vi "Thorlabs_CCS_Test_Panel.vi"() -> ()   [LabVIEW 2021]
doc: "Instrument test panel"
uses:
  _Controls/Thorlabs_CCS_Detector_Info.ctl
  _Controls/Thorlabs_CCS_Configuration.ctl
panel:
  out "XY Graph":T1(graph)
  in  "Tab Control":enum32{"Detector", "Configuration", "Capture"}(tab)
  out "Detector":T2
  in  "Connect":bool
  in  "USB VISA Resource Name":string="USB0::0x1313::0x8089::M00463105::RAW"
  in  "Auto detect USB devices":bool
  in  "Configuration":T3={"Acquisition_Mode"=enum."Continuos", "Trigger_Source"=enum."Auto/Internal", "Integration_Time_[s]"=0.5}
  out "Period [s]":dbl
  out "Counter":i32
  in  "NbrLines":i32=-1 caption="NbrLines\n(-1=endless)" min=-2 max=1000000
  in  "Capture":bool
  out "# elements in queue":i32
  out "Error Message":string caption="Error Description"
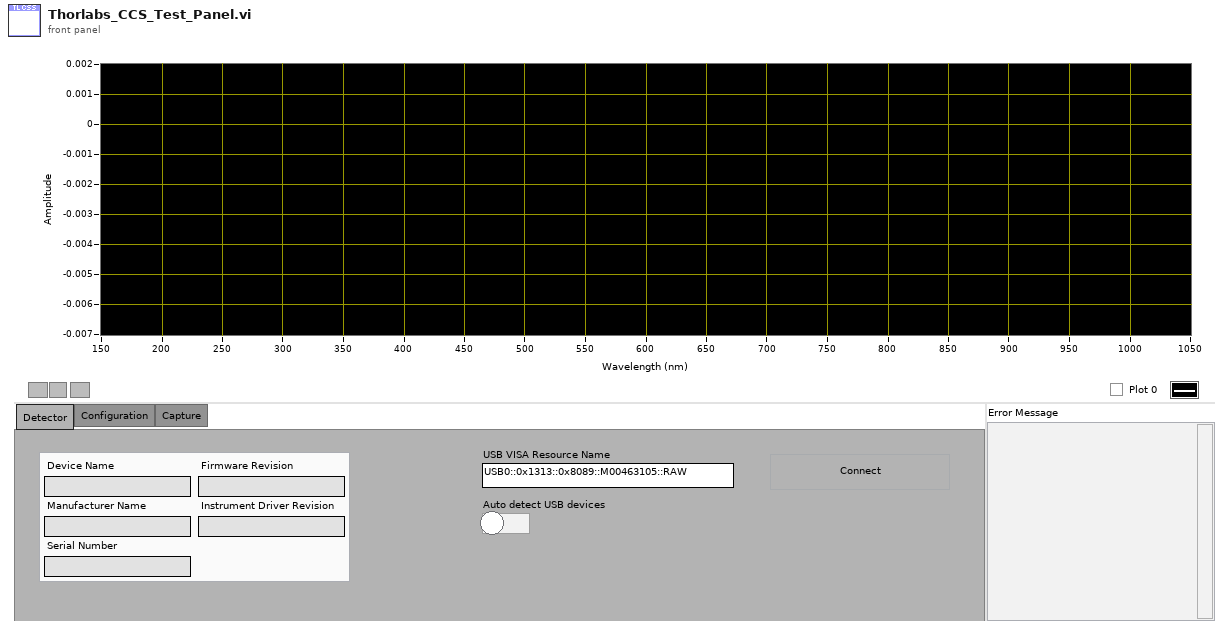
[diagram p1: front panel]
types:
  T1 = cluster{"Wavelength Data Array":dbl[], "Data":dbl[]}
  T2 = typedef "Thorlabs_CCS_Detector_Info.ctl" = cluster{"Device Name":string, "Manufacturer Name":string, "Serial Number":string, "Firmware Revision":string, "Instrument Driver Revision":string}
  T3 = typedef "Thorlabs_CCS_Configuration.ctl" = cluster{"Acquisition_Mode":enum16{"Single Scan", "Continuos"}, "Trigger_Source":enum16{"Auto/Internal", "External"}, "Integration_Time_[s]":dbl}
  T4 = cluster{"This VI":refnum<vi>, "Control":cluster{"Capture":refnum<vi>, "Tab Control":refnum<vi>, "NbrLines":refnum<vi>}, "Indicator":cluster{"Detector":refnum<vi>, "XY Graph":refnum<vi>}}
  T5 = enum32{"invalid app kind", "Development System", "Run Time System", "Student Edition", "Embedded LabVIEW", "Evaluation", "Custom"}
  T6 = enum8{"Enabled", "Disabled", "Disabled and Grayed Out"}
  T7 = enum32{"Page Enabled", "Page Disabled", "Page Disabled & Grayed"}
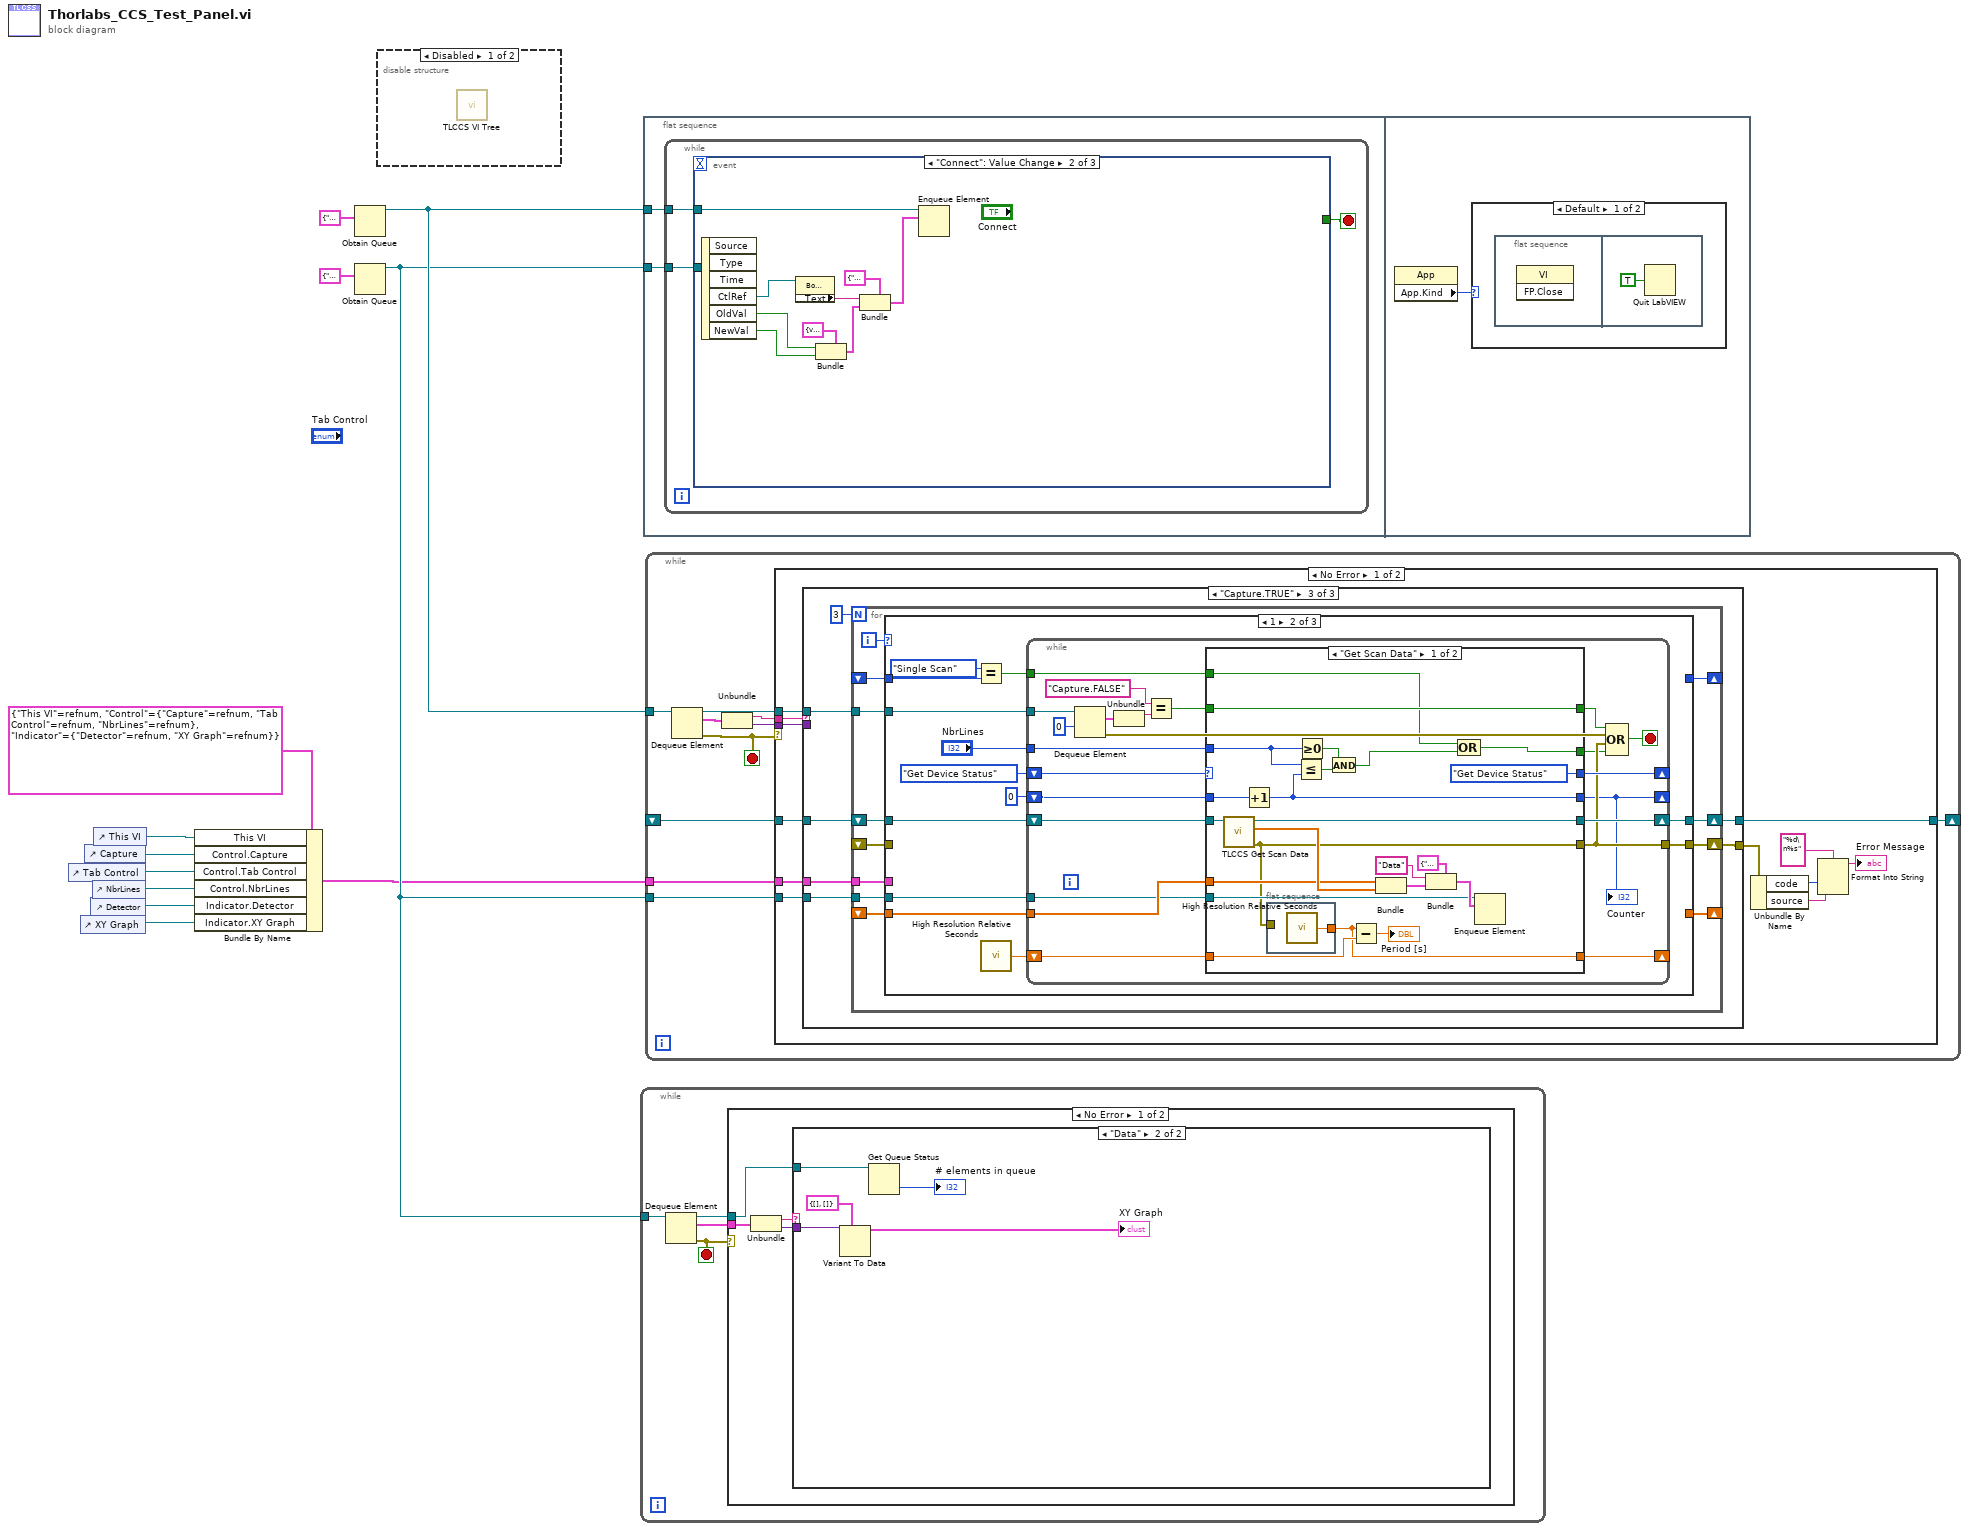
[diagram p0: block diagram]
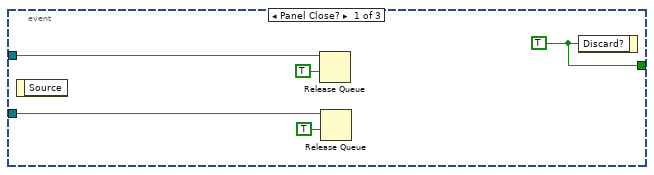
[diagram p5: hidden frame]
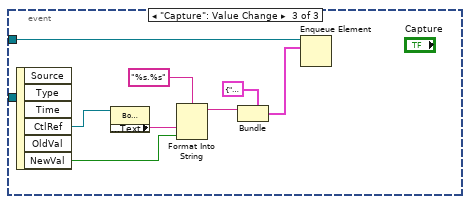
[diagram p6: hidden frame]
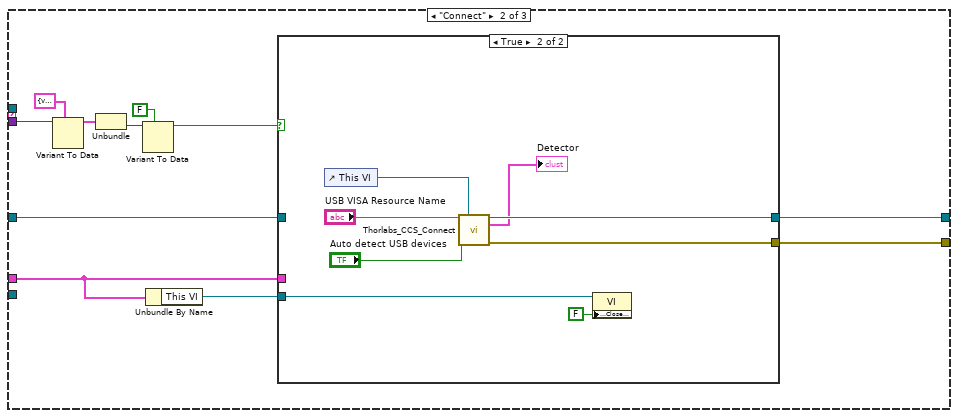
[diagram p9: hidden frame]
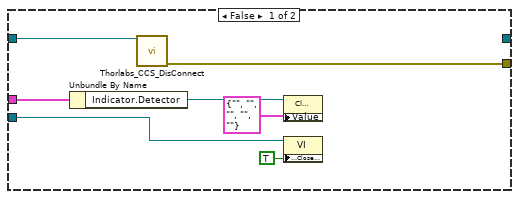
[diagram p10: hidden frame]
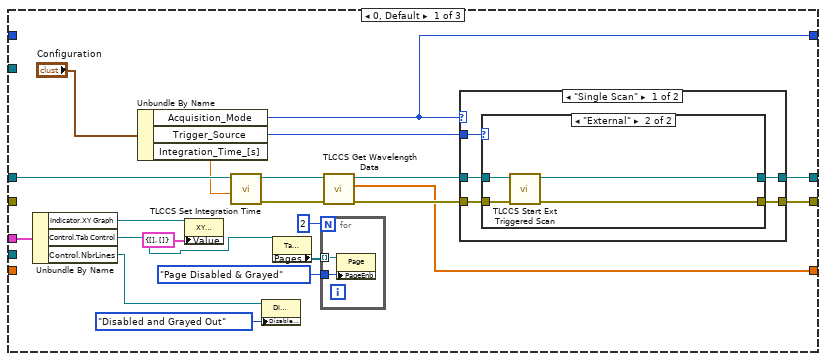
[diagram p11: hidden frame]
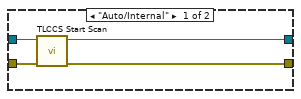
[diagram p12: hidden frame]
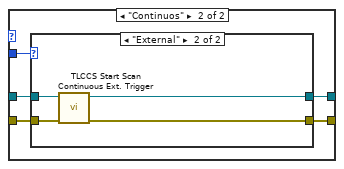
[diagram p13: hidden frame]
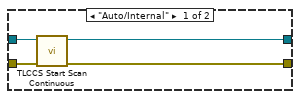
[diagram p14: hidden frame]
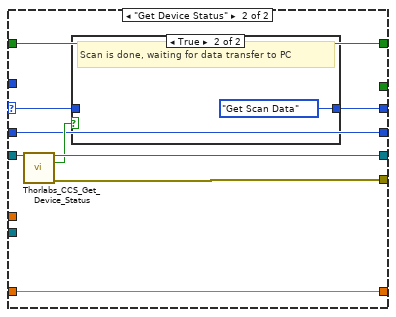
[diagram p15: hidden frame]
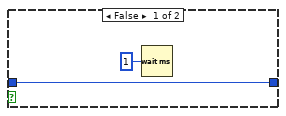
[diagram p16: hidden frame]
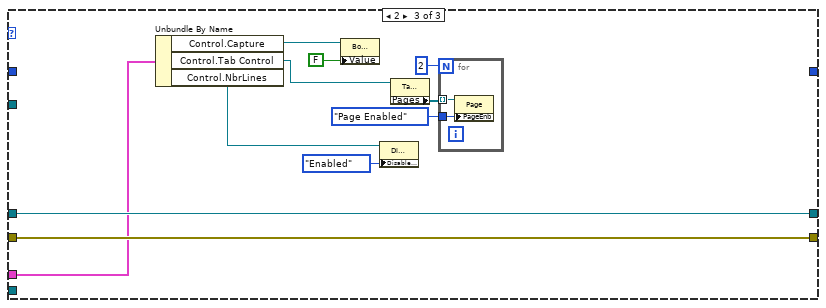
[diagram p17: hidden frame]
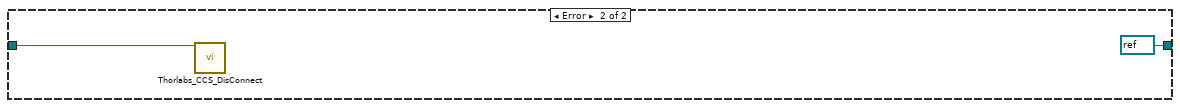
[diagram p18: hidden frame]
diagram:
  n1 = control-ref of="Tab Control"() -> (w5:refnum<vi>)
  n2 = control-ref of="XY Graph"() -> (w2:refnum<vi>)
  n3 = control-ref of="Capture"() -> (w7:refnum<vi>)
  n4 = control-ref of="Detector"() -> (w3:refnum<vi>)
  n5 = control-ref of="NbrLines"() -> (w4:refnum<vi>)
  n6 = control-ref of="This VI"() -> (w1:refnum<vi>)
  n7 = Bundle By Name(cluster=T4 {"This VI"=refnum, "Control"={"Capture"=refnum, "Tab Control"=refnum, "NbrLines"=refnum}, "Indicator"={"Detector"=refnum, "XY Graph"=refnum}}, "This VI"=w1, "Control.Capture"=w7, "Control.Tab Control"=w5, "Control.NbrLines"=w4, "Indicator.Detector"=w3, "Indicator.XY Graph"=w2) -> (w6:T4)
  n8 = Obtain Queue(element data type=cluster{"Command":string, "Data":variant} {"Command"="", "Data"=variant}) -> (queue out=w11:refnum<queue>)  [unwired: 4 in, 2 out]
  n9 = Obtain Queue(element data type=cluster{"Command":string, "Data":variant} {"Command"="", "Data"=variant}) -> (queue out=w9:refnum<queue>)  [unwired: 4 in, 2 out]
  n10 = disable-structure shown="Disabled" {
    frame Disabled {
      n11 = call <instrlib>:"TLCCS VI Tree.vi"() -> ()  [unwired: 12 in]
    }
    frame Enabled {
    }
  }
  n12 = while {
    tunnel: w9 -> [w16]
    stop <- w15 stop-if-true
    n13 = Dequeue Element(queue=w16) -> (queue out=w13:refnum<queue>, element=w14:cluster{"Command":string, "Data":variant}, error out=w15:errorcluster)  [unwired: 2 in, 1 out]
    n14 = case shown="No Error" w15 {
      tunnel: w14 -> [w20 _]
      tunnel: w13 -> [w17 _]
      frame No Error {
        n15 = Unbundle(w20) -> ("Command"=w19:string, "Data"=w18:variant)
        n16 = case shown="\"Data\"" w19 {
          tunnel: w18 -> [_ w23]
          tunnel: w17 -> [_ w25]
          frame Default {
          }
          frame "Data" {
            n17 = Variant To Data(type=T1 {"Wavelength Data Array"=[], "Data"=[]} ("cluster"), Variant=w23) -> (data=→"XY Graph":T1)  [unwired: 1 in, 1 out]
            n18 = Get Queue Status(queue=w25) -> (# elements in queue=→"# elements in queue":i32)  [unwired: 2 in, 7 out]
          }
        }
      }
      frame Error {
      }
    }
  }
  n19 = flat-sequence {
    tunnel: w11 -> [w27]
    tunnel: w9 -> [w26]
    frame #0 {
      n20 = while {
        tunnel: w27 -> [w30]
        tunnel: w26 -> [w28]
        stop <- w29 stop-if-true
        n21 = event shown="[1] \"Connect\": Value Change" {
          selector: _ -> [_ _ _]
          dyn-events: _ -> [_ _ _]
          timeout: _ -> [_ _ _]
          tunnel: w30 -> [w32 w39 w50]
          tunnel: [w35 _ _] -> w29
          tunnel: w28 -> [w31 _ _]
          event Panel Close? {
            w35 = TRUE ("Discard?")
            n22 = event-data() -> ()  [unwired: 1 in, 1 out]
            n23 = Release Queue(queue=w32, force destroy? (F)=TRUE) -> ()  [unwired: 1 in, 3 out]
            n24 = Release Queue(queue=w31, force destroy? (F)=TRUE) -> ()  [unwired: 1 in, 3 out]
            n25 = event-data("Discard?"=w35) -> ()  [unwired: 1 in, 1 out]
          }
          event "Connect": Value Change {
            n26 = event-data() -> ("CtlRef"=w38:refnum<vi>, "OldVal"=w37:bool, "NewVal"=w36:bool)  [unwired: 1 in, 3 out]
            n27 = property class="Bool (strict)"(reference=w38) -> ("Label.Text"=w43:string)  [unwired: 1 in, 2 out]
            n28 = Bundle(cluster=cluster{"OldVal":variant, "NewVal":variant} {"OldVal"=variant, "NewVal"=variant}, "OldVal"=w37, "NewVal"=w36) -> (w41:cluster{"OldVal":variant, "NewVal":variant})
            n29 = Bundle(cluster=cluster{"Command":string, "Data":variant} {"Command"="", "Data"=variant} ("element"), "Command"=w43, "Data"=w41) -> (w40:cluster{"Command":string, "Data":variant})
            n30 = Enqueue Element(queue=w39, element=w40) -> ()  [unwired: 2 in, 3 out]
          }
          event "Capture": Value Change {
            n31 = event-data() -> ("CtlRef"=w49:refnum<vi>, "NewVal"=w47:bool)  [unwired: 1 in, 4 out]
            n32 = property class="Bool (strict)"(reference=w49) -> ("Label.Text"=w48:string)  [unwired: 1 in, 2 out]
            n33 = Format Into String(format string="%s.%s", w48, w47) -> (resulting string=w45:string)  [unwired: 2 in, 1 out]
            n34 = Bundle(cluster=cluster{"Command":string, "Data":variant} {"Command"="", "Data"=variant} ("element"), "Command"=w45) -> (w51:cluster{"Command":string, "Data":variant})  [unwired: 1 in]
            n35 = Enqueue Element(queue=w50, element=w51) -> ()  [unwired: 2 in, 3 out]
          }
        }
      }
    }
    frame #1 {
      n36 = property class="App"() -> ("App.Kind"=w53:T5)  [unwired: 2 in, 2 out]
      n37 = case shown="Default" w53 {
        frame Default {
          n38 = flat-sequence {
            frame #0 {
              n39 = invoke class="VI" method="FP.Close"() -> ()  [unwired: 3 in, 3 out]
            }
            frame #1 {
              n40 = Quit LabVIEW(quit? (T)=TRUE) -> ()
            }
          }
        }
        frame "Development System" {
        }
      }
    }
  }
  n41 = while {
    tunnel: w11 -> [w61]
    shift-right: [w64] -> _
    shift-left: _ -> [w63]
    tunnel: w6 -> [w62]
    tunnel: w9 -> [w55]
    stop <- w60 stop-if-true
    n42 = Dequeue Element(queue=w61) -> (queue out=w59:refnum<queue>, element=w58:cluster{"Command":string, "Data":variant}, error out=w60:errorcluster)  [unwired: 2 in, 1 out]
    n43 = Unbundle(w58) -> ("Command"=w57:string, "Data"=w56:variant)
    n44 = case shown="No Error" w60 {
      tunnel: w56 -> [w75 _]
      tunnel: w57 -> [w76 _]
      tunnel: w59 -> [w74 _]
      tunnel: [w73 refnum<visa-resource-name> refnum ("VISA Refnum out")] -> w64
      tunnel: w63 -> [w72 w258]
      tunnel: w62 -> [w66 _]
      tunnel: w55 -> [w65 _]
      frame No Error {
        n45 = case shown="\"Capture.TRUE\"" w76 {
          tunnel: w75 -> [_ w85 _]
          tunnel: w74 -> [_ _ w108]
          tunnel: [w77 w82 w109] -> w73
          tunnel: w72 -> [w77 w80 w110]
          tunnel: [_ w81 w105] -> w67
          tunnel: w66 -> [_ w78 w104]
          tunnel: w65 -> [_ _ w107]
          frame Default {
          }
          frame "Connect" {
            n46 = Variant To Data(type=cluster{"OldVal":variant, "NewVal":variant} {"OldVal"=variant, "NewVal"=variant} ("cluster"), Variant=w85) -> (data=w88:cluster{"OldVal":variant, "NewVal":variant})  [unwired: 1 in, 1 out]
            n47 = Unbundle(w88) -> ("NewVal"=w87:variant)  [unwired: 1 out]
            n48 = Variant To Data(type=FALSE, Variant=w87) -> (data=w83:bool)  [unwired: 1 in, 1 out]
            n49 = Unbundle By Name(w78) -> ("This VI"=w79:refnum<vi>)
            n50 = case shown="True" w83 {
              tunnel: [_ w103] -> w82
              tunnel: [w94 w102] -> w81
              tunnel: w80 -> [w95 _]
              tunnel: w78 -> [w93 _]
              tunnel: w79 -> [w89 w98]
              frame False {
                n51 = Unbundle By Name(w93) -> ("Indicator.Detector"=w92:refnum<vi>)
                n52 = call "Thorlabs_CCS_DisConnect.vi"("VISA Refnum in"=w95) -> ("error out"=w94:errorcluster)  [unwired: 14 in]
                n53 = property class="Clust (strict)"(reference=w92, "Value"=T2 {"Device Name"="", "Manufacturer Name"="", "Serial Number"="", "Firmware Revision"="", "Instrument Driver Revision"=""}) -> ()  [unwired: 1 in, 2 out]
                n54 = property class="VI"(reference=w89, "Front Panel.Closeable"=TRUE ("Front Panel Window:Closeable")) -> ()  [unwired: 1 in, 2 out]
              }
              frame True {
                n55 = control-ref of="This VI"() -> (w100:refnum<vi>)
                n56 = call "Thorlabs_CCS_Connect.vi"("USB VISA Resource Name"="USB VISA Resource Name", "Top VI reference"=w100, "Auto detect USB devices"="Auto detect USB devices") -> ("Instrument Refnum"=w103:refnum<visa-resource-name>, "Detector"=→"Detector":T2, "error out"=w102:errorcluster)  [unwired: 10 in]
                n57 = property class="VI"(reference=w98, "Front Panel.Closeable"=FALSE ("Front Panel Window:Closeable")) -> ()  [unwired: 1 in, 2 out]
              }
            }
          }
          frame "Capture.TRUE" {
            n58 = for {
              N: 3 -> [_]
              shift-right: [w120] -> w109
              shift-left: w110 -> [w121]
              tunnel: w108 -> [w118]
              shift-right: [w117] -> _
              shift-left: _ -> [w116]
              tunnel: w107 -> [w115]
              shift-right: [w119] -> w105
              shift-left: _ -> [w114]
              tunnel: w104 -> [w113]
              shift-right: [w112] -> _
              shift-left: _ -> [w111]
              i -> [w122]
              n59 = case shown="1" w122 {
                tunnel: w121 -> [w141 w183 w254]
                tunnel: [w135 w182 w254] -> w120
                tunnel: [w134 w180 w253] -> w119
                tunnel: w118 -> [_ w184 _]
                tunnel: [w133 _ _] -> w117
                tunnel: w116 -> [_ w179 _]
                tunnel: w115 -> [_ w178 _]
                tunnel: w114 -> [_ _ w253]
                tunnel: w113 -> [w131 _ w252]
                tunnel: [w132 _ _] -> w112
                tunnel: w111 -> [_ w174 _]
                frame 0, Default {
                  n60 = Unbundle By Name(w131) -> ("Indicator.XY Graph"=w130:refnum<vi>, "Control.Tab Control"=w124:refnum<vi>, "Control.NbrLines"=w123:refnum<vi>)
                  n61 = Unbundle By Name("Configuration") -> ("Acquisition_Mode"=w132:enum16{"Single Scan", "Continuos"}, "Trigger_Source"=w136:enum16{"Auto/Internal", "External"}, "Integration_Time_[s]"=w139:dbl)
                  n62 = property class="XYGraph (strict)"(reference=w130, "Value"=T1 {"Wavelength Data Array"=[], "Data"=[]}) -> ()  [unwired: 1 in, 2 out]
                  n63 = call <instrlib>:"TLCCS Set Integration Time.vi"("Integration Time [s] (0.001)"=w139, "instrument handle"=w141) -> ("error out"=w142:errorcluster, "instrument handle out"=w143:refnum<visa-resource-name>)  [unwired: 8 in]
                  n64 = property class="DigNum (strict)"(reference=w123, "DisabledEnum"=T6."Disabled and Grayed Out" ("Disabled")) -> ()  [unwired: 1 in, 2 out]
                  n65 = property class="TabCtl (strict)"(reference=w124) -> ("Pages"=w128:refnum<vi>[])  [unwired: 1 in, 2 out]
                  n66 = for {
                    N: 2 -> [_]
                    tunnel: w128 -> [w145] mode=indexing
                    tunnel: T7."Page Disabled & Grayed" ("Page Enabled State") -> [w144]
                    n67 = property class="Page"(reference=w145, "PageEnb"=w144) -> ()  [unwired: 1 in, 2 out]
                  }
                  n68 = call <instrlib>:"TLCCS Get Wavelength Data.vi"("error in (no error)"=w142, "instrument handle"=w143) -> ("error out"=w138:errorcluster, "Wavelength Data Array"=w133:dbl[], "instrument handle out"=w137:refnum<visa-resource-name>)  [unwired: 5 in, 2 out]
                  n69 = case shown="\"Single Scan\"" w132 {
                    tunnel: w138 -> [w149 w162]
                    tunnel: w137 -> [w150 w163]
                    tunnel: w136 -> [w146 w159]
                    tunnel: [w148 w161] -> w134
                    tunnel: [w147 w160] -> w135
                    frame "Single Scan" {
                      n70 = case shown="\"External\"" w146 {
                        tunnel: w150 -> [w154 w158]
                        tunnel: w149 -> [w153 w157]
                        tunnel: [w152 w156] -> w148
                        tunnel: [w151 w155] -> w147
                        frame "Auto/Internal" {
                          n71 = call <instrlib>:"TLCCS Start Scan.vi"("error in (no error)"=w153, "instrument handle"=w154) -> ("error out"=w152:errorcluster, "instrument handle out"=w151:refnum<visa-resource-name>)  [unwired: 8 in]
                        }
                        frame "External" {
                          n72 = call <instrlib>:"TLCCS Start Ext Triggered Scan.vi"("error in (no error)"=w157, "instrument handle"=w158) -> ("error out"=w156:errorcluster, "instrument handle out"=w155:refnum<visa-resource-name>)  [unwired: 8 in]
                        }
                      }
                    }
                    frame "Continuos" {
                      n73 = case shown="\"External\"" w159 {
                        tunnel: w163 -> [w167 w171]
                        tunnel: w162 -> [w166 w170]
                        tunnel: [w165 w169] -> w161
                        tunnel: [w164 w168] -> w160
                        frame "Auto/Internal" {
                          n74 = call <instrlib>:"TLCCS Start Scan Continuous.vi"("error in (no error)"=w166, "instrument handle"=w167) -> ("error out"=w165:errorcluster, "instrument handle out"=w164:refnum<visa-resource-name>)  [unwired: 8 in]
                        }
                        frame "External" {
                          n75 = call <instrlib>:"TLCCS Start Scan Continuous Ext. Trigger.vi"("error in (no error)"=w170, "instrument handle"=w171) -> ("error out"=w169:errorcluster, "instrument handle out"=w168:refnum<visa-resource-name>)  [unwired: 8 in]
                        }
                      }
                    }
                  }
                }
                frame 1 {
                  n76 = Equal?(x=enum16{"Single Scan", "Continuos"}."Single Scan", y=w174) -> (x = y?=w172:bool)
                  n77 = call <vilib>:"High Resolution Relative Seconds.vi"() -> ("relative seconds"=w175:dbl)
                  n78 = while {
                    tunnel: w184 -> [w202]
                    shift-right: [w205] -> w182
                    shift-left: w183 -> [w207]
                    shift-right: [w204] -> _
                    shift-left: enum16{"Get Device Status", "Get Scan Data"}."Get Device Status" -> [w206]
                    tunnel: [w198] -> w180
                    tunnel: w179 -> [w193]
                    tunnel: w178 -> [w192]
                    shift-right: [w190] -> _
                    shift-left: 0 -> [w191]
                    tunnel: "NbrLines" -> [w188]
                    shift-right: [w186] -> _
                    shift-left: w175 -> [w187]
                    tunnel: w172 -> [w185]
                    stop <- w197 stop-if-true
                    n79 = Dequeue Element(queue=w202, timeout in ms (-1)=0) -> (element=w203:cluster{"Command":string, "Data":variant}, error out=w196:errorcluster)  [unwired: 1 in, 2 out]
                    n80 = Unbundle(w203) -> ("Command"=w200:string)  [unwired: 1 out]
                    n81 = Equal?(x="Capture.FALSE", y=w200) -> (x = y?=w195:bool)
                    n82 = case shown="\"Get Scan Data\"" w206 {
                      selector: w206 -> [_ w236]
                      tunnel: w207 -> [w229 w240]
                      tunnel: [w228 w239] -> w205
                      tunnel: [w210 w238] -> w198
                      tunnel: [enum16{"Get Device Status", "Get Scan Data"}."Get Device Status" w235] -> w204
                      tunnel: w195 -> [w227 w233]
                      tunnel: [w227 w233] -> w194
                      tunnel: w193 -> [w221 _]
                      tunnel: w192 -> [w220 _]
                      tunnel: w191 -> [w217 w234]
                      tunnel: [w216 w234] -> w190
                      tunnel: [w209 _] -> w189
                      tunnel: w188 -> [w214 _]
                      tunnel: w187 -> [w212 w232]
                      tunnel: [w211 w232] -> w186
                      tunnel: w185 -> [w208 _]
                      frame "Get Scan Data" {
                        n83 = call <instrlib>:"TLCCS Get Scan Data.vi"("instrument handle"=w229) -> ("error out"=w210:errorcluster, "Data"=w222:dbl[], "instrument handle out"=w228:refnum<visa-resource-name>)  [unwired: 8 in]
                        n84 = Increment(x=w217) -> (x+1=w216:i32)
                        n85 = flat-sequence {
                          tunnel: [w231] -> w211
                          tunnel: w210 -> [_]
                          frame #0 {
                            n86 = call <vilib>:"High Resolution Relative Seconds.vi"() -> ("relative seconds"=w231:dbl)
                          }
                        }
                        n87 = Less Or Equal?(x=w214, y=w216) -> (x <= y?=w219:bool)
                        n88 = Greater Or Equal To 0?(x=w214) -> (x >= 0?=w218:bool)
                        n89 = And(x=w218, y=w219) -> (x .and. y?=w215:bool)
                        n90 = Subtract(x=w211, y=w212) -> (x-y=→"Period [s]":dbl)
                        n91 = Bundle("Wavelength Data Array"=w221, "Data"=w222) -> (w223:T1)  [unwired: 1 in]
                        n92 = Bundle(cluster=cluster{"Command":string, "Data":variant} {"Command"="", "Data"=variant} ("element"), "Command"="Data", "Data"=w223) -> (w225:cluster{"Command":string, "Data":variant})
                        n93 = Compound Arithmetic op=OR(w208, w215) -> (w209:bool)
                        n94 = Enqueue Element(queue=w220, element=w225) -> ()  [unwired: 2 in, 3 out]
                      }
                      frame "Get Device Status" {
                        n95 = call "Thorlabs_CCS_Get_Device_Status.vi"("VISA Refnum in"=w240) -> ("VISA Refnum out"=w239:refnum<visa-resource-name>, "Scan is done"=w237:bool, "error out"=w238:errorcluster)  [unwired: 12 in]
                        n96 = case shown="True" w237 {
                          tunnel: w236 -> [w242 _]
                          tunnel: [w242 enum16{"Get Device Status", "Get Scan Data"}."Get Scan Data"] -> w235
                          frame False {
                            n97 = Wait (ms)(milliseconds to wait=u32 1) -> ()  [unwired: 1 out]
                          }
                          frame True {
                            # "Scan is done, waiting for data transfer to PC"
                          }
                        }
                      }
                    }
                    "Counter" <- w190
                    n98 = Compound Arithmetic op=OR(w194, w196, w198, w189) -> (w197:bool)
                  }
                }
                frame 2 {
                  n99 = Unbundle By Name(w252) -> ("Control.Capture"=w251:refnum<vi>, "Control.Tab Control"=w245:refnum<vi>, "Control.NbrLines"=w244:refnum<vi>)
                  n100 = property class="Bool (strict)"(reference=w251, "Value"=FALSE) -> ()  [unwired: 1 in, 2 out]
                  n101 = property class="DigNum (strict)"(reference=w244, "DisabledEnum"=T6."Enabled" ("Disabled")) -> ()  [unwired: 1 in, 2 out]
                  n102 = property class="TabCtl (strict)"(reference=w245) -> ("Pages"=w249:refnum<vi>[])  [unwired: 1 in, 2 out]
                  n103 = for {
                    N: 2 -> [_]
                    tunnel: w249 -> [w256] mode=indexing
                    tunnel: T7."Page Enabled" ("Page Enabled State") -> [w255]
                    n104 = property class="Page"(reference=w256, "PageEnb"=w255) -> ()  [unwired: 1 in, 2 out]
                  }
                }
              }
            }
          }
        }
        n105 = Unbundle By Name(w67) -> ("code"=w70:i32, "source"=w69:string)
        n106 = Format Into String(format string="%d\n%s", w70, w69) -> (resulting string=→"Error Message":string)  [unwired: 2 in, 1 out]
      }
      frame Error {
        n107 = call "Thorlabs_CCS_DisConnect.vi"("VISA Refnum in"=w258) -> ()  [unwired: 14 in, 1 out]
      }
    }
  }
